vi "Read ABCFirstKickerRole.vi"(8 "error in (no error)":errorcluster, 11 "Rolebook in":refnum<class "Rolebook.lvclass">) -> (0 "error out":errorcluster, 2 "ABCFirstKickerRole":refnum<class "ABCFirstKickerRole.lvclass">, 3 "Rolebook out":refnum<class "Rolebook.lvclass">)   [LabVIEW 2023, in "Rolebook.lvclass"]
uses:
  Rolebook.lvclass
  ABCFirstKickerRole_class/ABCFirstKickerRole.lvclass
  Rolebook.lvclass/Rolebook.ctl
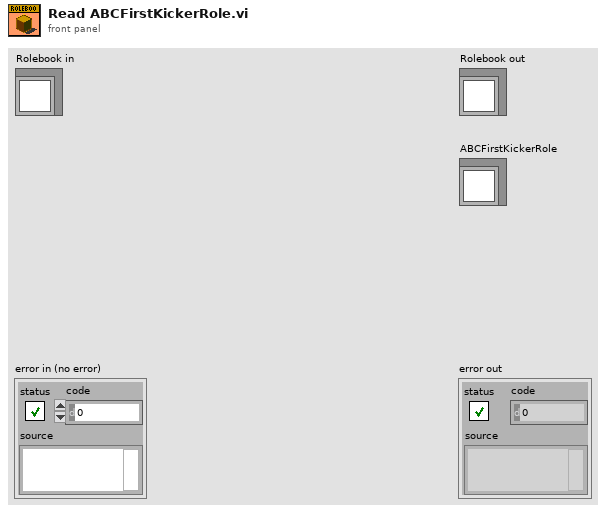
[diagram p1: front panel]
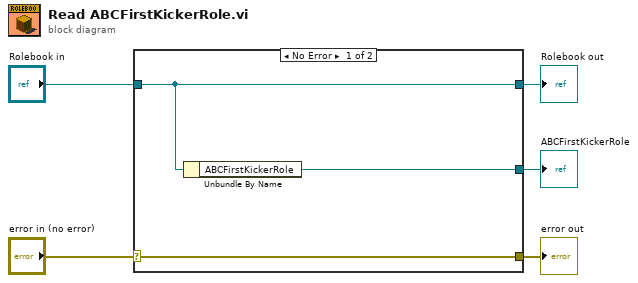
[diagram p0: block diagram]
diagram:
  n1 = case shown="No Error" "error in (no error)" {
    selector: "error in (no error)" -> [w8 w9]
    tunnel: [w8 w9] -> w4
    tunnel: [w7 w10] -> w2
    tunnel: "Rolebook in" -> [w7 w10]
    tunnel: [w6 _] -> w1
    frame No Error {
      n2 = Unbundle By Name(w7) -> ("ABCFirstKickerRole"=w6:refnum<class "ABCFirstKickerRole.lvclass">)
    }
    frame Error {
    }
  }
  "error out" <- w4
  "Rolebook out" <- w2
  "ABCFirstKickerRole" <- w1
